vi "verify_laser_alignment.vi"() -> (0 "error out":errorcluster)   [LabVIEW 2018]
doc: "Turn On Power Supply\nChannel 1: 12V, 8A\nChannel 2: 12V, 2A"
panel:
  in  "error in (no error)":errorcluster
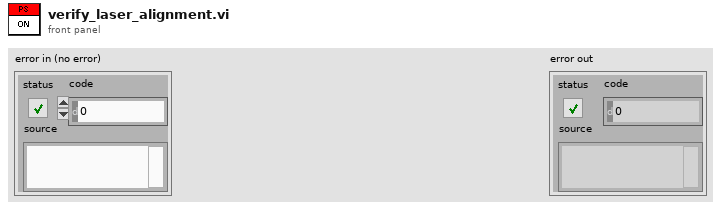
[diagram p1: front panel]
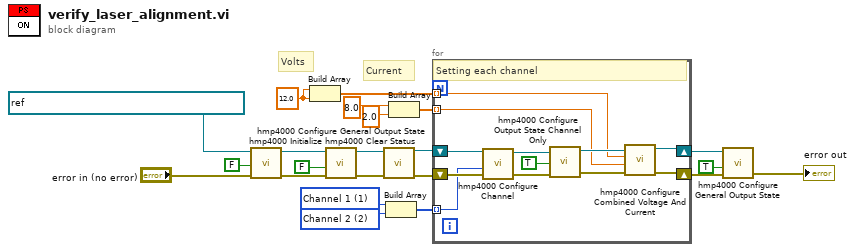
[diagram p0: block diagram]
diagram:
  w10 = 2 items=["Channel 1"=1, "Channel 2"=2, "Channel 3"=3, "Channel 4"=4] ("Channel (Channel 1)")
  w11 = 1 items=["Channel 1"=1, "Channel 2"=2, "Channel 3"=3, "Channel 4"=4] ("Channel (Channel 1)")
  w4 = 12.0 ("element")
  # "Current"
  # "Volts"
  n1 = call "hmp4000 Initialize.vi"("error in (no error)"="error in (no error)", "Reset (T: Reset)"=FALSE, "VISA resource name"=refnum<visa-resource-name> "TCPIP::10.42.0.201::5025::SOCKET") -> ("error out"=w19:errorcluster, "VISA resource name out"=w20:refnum<visa-resource-name>)  [unwired: 7 in]
  n2 = Build Array(w4, w4) -> (w15:dbl[])
  n3 = call "hmp4000 Configure General Output State.vi"("error in (no error)"=w19, "Output State (Off)"=FALSE, "VISA resource name"=w20) -> ("error out"=w8:errorcluster, "VISA resource name out"=w7:refnum<visa-resource-name>)  [unwired: 7 in]
  n4 = call "hmp4000 Clear Status.vi"("VISA resource name"=w7, "error in (no error)"=w8) -> ("VISA resource name out"=w6:refnum<visa-resource-name>, "error out"=w5:errorcluster)  [unwired: 12 in]
  n5 = Build Array(w11, w10) -> (w9:i32[])
  n6 = Build Array(8.0 ("element"), 2.0 ("element")) -> (w14:dbl[])
  n7 = for {
    shift-right: [w27] -> w21
    shift-left: w5 -> [w30]
    shift-right: [w26] -> w22
    shift-left: w6 -> [w31]
    tunnel: w15 -> [w25] mode=indexing
    tunnel: w14 -> [w24] mode=indexing
    tunnel: w9 -> [w23] mode=indexing
    # "Setting each channel"
    n8 = call "hmp4000 Configure Channel.vi"("error in (no error)"=w30, "Channel (Channel 1)"=w23, "VISA resource name"=w31) -> ("error out"=w33:errorcluster, "VISA resource name out"=w32:refnum<visa-resource-name>)  [unwired: 7 in]
    n9 = call "hmp4000 Configure Output State Channel Only.vi"("error in (no error)"=w33, "Output State (Off)"=TRUE ("t"), "VISA resource name"=w32) -> ("error out"=w28:errorcluster, "VISA resource name out"=w29:refnum<visa-resource-name>)  [unwired: 7 in]
    n10 = call "hmp4000 Configure Combined Voltage And Current.vi"("error in (no error)"=w28, "Current (0.0)"=w24, "Voltage (0.0)"=w25, "VISA resource name"=w29) -> ("error out"=w27:errorcluster, "VISA resource name out"=w26:refnum<visa-resource-name>)  [unwired: 6 in]
  }
  n11 = call "hmp4000 Configure General Output State.vi"("error in (no error)"=w21, "Output State (Off)"=TRUE, "VISA resource name"=w22) -> ("error out"=→"error out":errorcluster)  [unwired: 7 in, 1 out]
